vi "sub_msgbox.vi"(11 "Reference pid values":string) -> ()   [LabVIEW 2019]
panel:
  in  "STOP":bool
  out "bg":bool
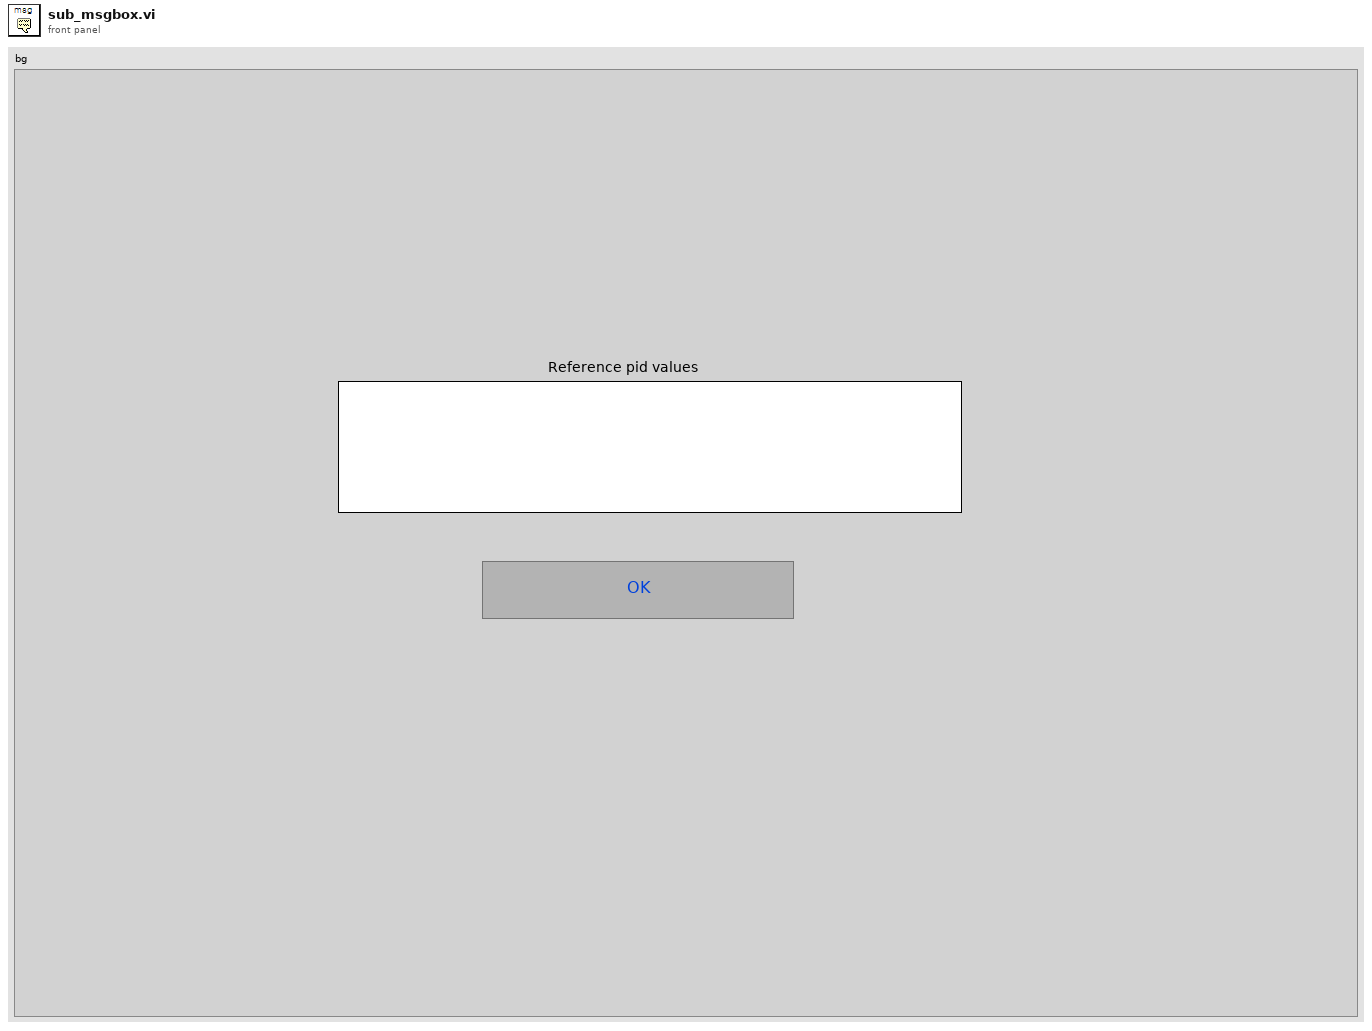
[diagram p1: front panel]
types:
  T1 = enum32{"Invalid", "Standard", "Closed", "Hidden", "Minimized", "Maximized"}
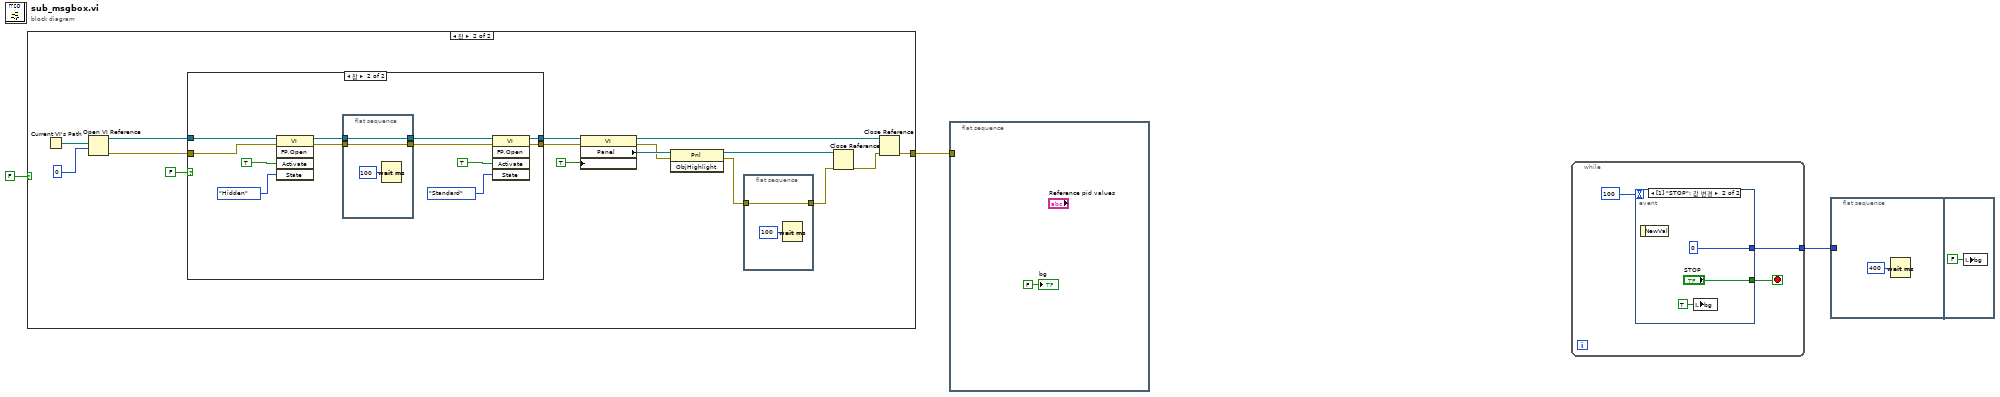
[diagram p0: block diagram]
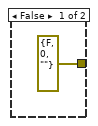
[diagram p2: hidden frame]
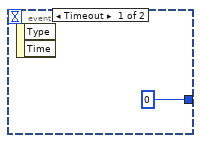
[diagram p4: hidden frame]
diagram:
  n1 = case shown="참" FALSE {
    tunnel: [errorcluster {"status"=FALSE, "code"=0, "source"=""} ("error out") w15] -> w3
    frame False {
    }
    frame True {
      n2 = Current VI's Path() -> (path=w16:path)
      n3 = Open VI Reference(vi path=w16, options=0 ("옵션")) -> (vi reference=w6:refnum<vi>, error out=w7:errorcluster)  [unwired: 4 in]
      n4 = case shown="참" FALSE {
        tunnel: [w21 w32] -> w9
        tunnel: [w22 w31] -> w8
        tunnel: w7 -> [w21 w28]
        tunnel: w6 -> [w22 w27]
        frame False {
        }
        frame True {
          n5 = invoke class="VI" method="FP.Open"(reference=w27, error in=w28, "Activate"=TRUE, "State"=T1."Hidden") -> (reference out=w23:refnum<vi>, error out=w26:errorcluster)  [unwired: 1 in, 3 out]
          n6 = flat-sequence {
            tunnel: w26 -> [w37]
            tunnel: [w37] -> w25
            tunnel: [w35] -> w24
            tunnel: w23 -> [w35]
            frame #0 {
              n7 = Wait (ms)(milliseconds to wait=u32 100 ("대기 시간(ms)")) -> ()  [unwired: 1 out]
            }
          }
          n8 = invoke class="VI" method="FP.Open"(reference=w24, error in=w25, "Activate"=TRUE, "State"=T1."Standard") -> (reference out=w31:refnum<vi>, error out=w32:errorcluster)  [unwired: 1 in, 3 out]
        }
      }
      n9 = property class="VI"(reference=w8, error in=w9, "Front Panel.IsFrontmost"=TRUE ("프런트패널 윈도우:맨 앞으로")) -> (reference out=w19:refnum<vi>, error out=w17:errorcluster, "Panel"=w18:refnum<vi>)
      n10 = invoke class="Pnl" method="ObjHighlight"(reference=w18, error in=w17) -> (reference out=w14:refnum<vi>, error out=w13:errorcluster)  [unwired: 1 in, 1 out]
      n11 = flat-sequence {
        tunnel: w13 -> [w39]
        tunnel: [w39] -> w12
        frame #0 {
          n12 = Wait (ms)(milliseconds to wait=u32 100 ("대기 시간(ms)")) -> ()  [unwired: 1 out]
        }
      }
      n13 = Close Reference(reference=w14, error in (no error)=w12) -> (error out=w11:errorcluster)
      n14 = Close Reference(reference=w19, error in (no error)=w11) -> (error out=w15:errorcluster)
    }
  }
  n15 = flat-sequence {
    tunnel: w3 -> [_]
    frame #0 {
      "bg" <- FALSE ("bg")
    }
  }
  n16 = while {
    tunnel: [w41] -> w1
    stop <- w43 stop-if-true
    n17 = event shown="[1] \"STOP\": 값 변경" {
      selector: _ -> [_ _]
      dyn-events: _ -> [_ _]
      timeout: 100 -> [_ _]
      tunnel: [_ "STOP"] -> w43
      tunnel: [u32 0 u32 0] -> w41
      event Timeout {
        n18 = event-data() -> ()  [unwired: 1 in, 2 out]
      }
      event "STOP": Value Change {
        n19 = event-data() -> ()  [unwired: 1 in, 1 out]
        n20 = local write "bg"(TRUE ("bg")) -> ()
      }
    }
  }
  n21 = flat-sequence {
    tunnel: w1 -> [_]
    frame #0 {
      n22 = Wait (ms)(milliseconds to wait=u32 400) -> ()  [unwired: 1 out]
    }
    frame #1 {
      n23 = local write "bg"(FALSE ("bg")) -> ()
    }
  }
